vi "Read Zone Name.vi"(8 "error in (no error)":errorcluster, 11 "Zone in":refnum<class "Zone.lvclass">) -> (0 "error out":errorcluster, 2 "Zone Name":string, 3 "Zone out":refnum<class "Zone.lvclass">)   [LabVIEW 2017, in "Zone.lvclass"]
uses:
  Zone.lvclass
  Zone.lvclass/Zone.ctl
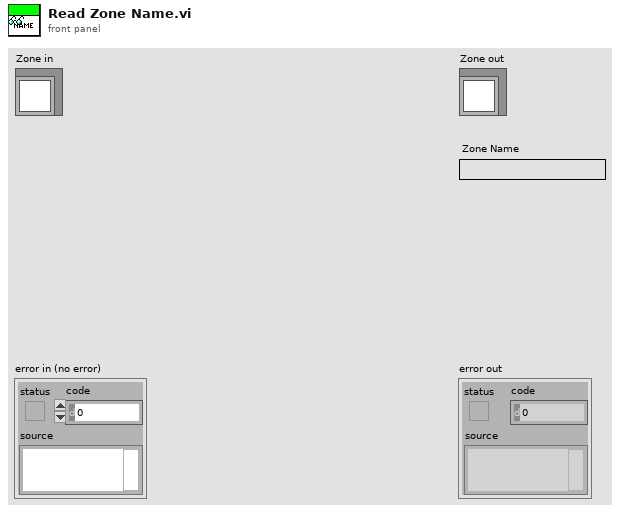
[diagram p1: front panel]
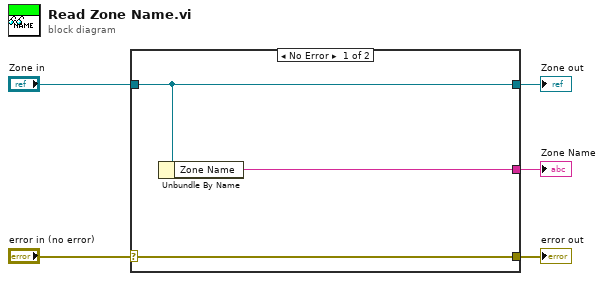
[diagram p0: block diagram]
diagram:
  n1 = case shown="No Error" "error in (no error)" {
    selector: "error in (no error)" -> [w8 w9]
    tunnel: [w8 w9] -> w4
    tunnel: [w7 w10] -> w2
    tunnel: "Zone in" -> [w7 w10]
    tunnel: [w6 _] -> w1
    frame No Error {
      n2 = Unbundle By Name(w7) -> ("Zone Name"=w6:string)
    }
    frame Error {
    }
  }
  "error out" <- w4
  "Zone out" <- w2
  "Zone Name" <- w1
